vi "Constant iniPathSampleTypeEnum.vi"() -> (0 "appended path":path)   [LabVIEW 2018]
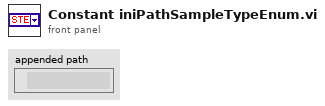
[diagram p1: front panel]
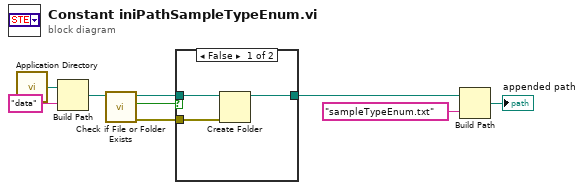
[diagram p0: block diagram]
diagram:
  n1 = call <vilib>:"Application Directory.vi"() -> ("Application Directory"=w7:path)
  n2 = Build Path(base path=w7, name or relative path="data") -> (appended path=w5:path)
  n3 = call <vilib>:"Check if File or Folder Exists.vi"("path"=w5) -> ("error out"=w2:errorcluster, "file or folder exists?"=w4:bool, "dup path"=w3:path)  [unwired: 8 in]
  n4 = case shown="False" w4 {
    tunnel: w3 -> [w12 w13]
    tunnel: w2 -> [w11 _]
    tunnel: [w10 w13] -> w1
    frame False {
      n5 = Create Folder(path (use dialog)=w12, error in=w11) -> (created path=w10:path)  [unwired: 1 in, 2 out]
    }
    frame True {
    }
  }
  n6 = Build Path(base path=w1, name or relative path="sampleTypeEnum.txt") -> (appended path=→"appended path":path)
